vi "modbus_rtu.vi"() -> ()   [LabVIEW 2020]
uses:
  <vilib>/Plasmionique/MB Master/MB_Master/MB_Master.lvclass
  <vilib>/Plasmionique/MB Master/MB_ADU/MB_ADU.lvclass/MB_ADU.ctl
  <vilib>/Plasmionique/MB Master/MB_ADU/Read TX Data.vi
  <vilib>/Plasmionique/MB Master/MB_ADU/Read RX Data.vi
  <vilib>/Plasmionique/MB Master/MB_ADU/Read RX Timestamp.vi
  <vilib>/Plasmionique/MB Master/MB_Master_Serial/MB_Master_Serial.lvclass
  C:/Program Files/National Instruments/LabVIEW 2020/vi.lib/Plasmionique/MB Master/MB_Master/MB_Master.lvclass
  <vilib>/Plasmionique/MB Master/MB_ADU/MB_ADU.lvclass
  <vilib>/Plasmionique/MB Master/MB Master.lvlib
panel:
  in  "Tab Control 2":enum32{"Comm Settings", "Comm Status"}(tab)
  in  "Open":bool
  in  "Close":bool
  in  "Poll Period (ms)":i32=100
  in  "COM Port":refnum<visa-resource-name>
  in  "Mode":enum16{"RTU", "ASCII"}(ring)
  in  "Slave Address":u8=1
  in  "Baud Rate (bps)":u32(ring)=19200 items=["9600"=9600, "19200"=19200, "38400"=38400, "57600"=57600, "115200"=115200, "460800"=460800, "921600"=921600]
  in  "Stop Bits":u16(ring)=10 items=["1.0"=10, "1.5"=15, "2.0"=20]
  in  "Parity":u16(ring) items=["None", "Odd", "Even", "Mark", "Space"]
  in  "Flow Control":u16(ring) items=["None", "XON/XOFF", "RTS/CTS", "XON/XOFF & RTS/CTS", "DTR/DSR", "XON/XOFF & DTR/DSR"]
  in  "Timeout (ms)":u32=300
  in  "Retries":i32=1
  out "Last Error Status":errorcluster
  out "Last RX":string
  out "Last TX":string
  out "Last RX Time":string
  out "Last Error Time":string
  out "dt (ms)":u32
  in  "IR Poll":bool
  in  "HR Poll":bool
  out "Open?":bool caption="Connected"
  in  "Write Hld Regs":bool
  in  "Read Hld Regs":bool
  in  "Read In Regs":bool
  in  "HR QTY":u16=1 caption="Quantity"
  in  "HR SA":u16 caption="Starting Address"
  in  "Holding Registers":u16[](array[numeric])
  in  "IR QTY":u16=1 caption="Quantity"
  in  "IR SA":u16 caption="Starting Address"
  out "Input Registers":u16[](array[numeric])
  # "Communication Settngs"
  # "Communication Status"
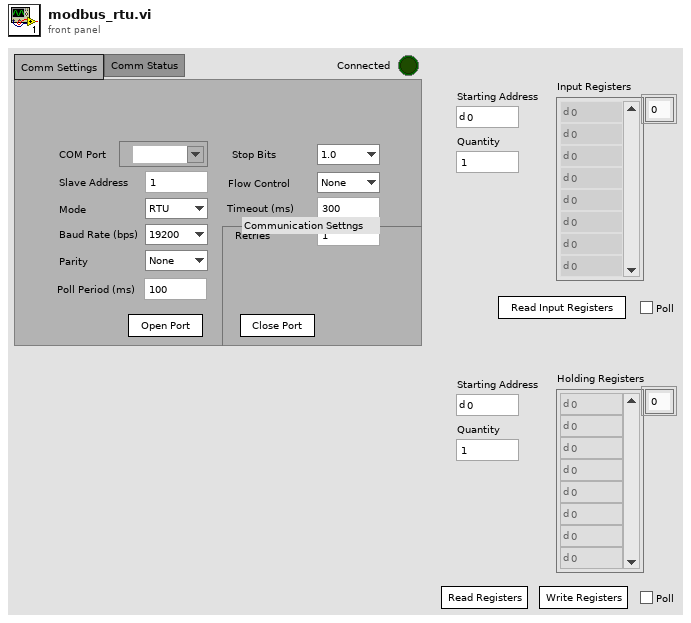
[diagram p1: front panel]
types:
  T1 = cluster{"baud rate (bps)":u32, "stop bits":u16, "parity":u16, "flow control":u16, "timeout":u32, "retries":i32}
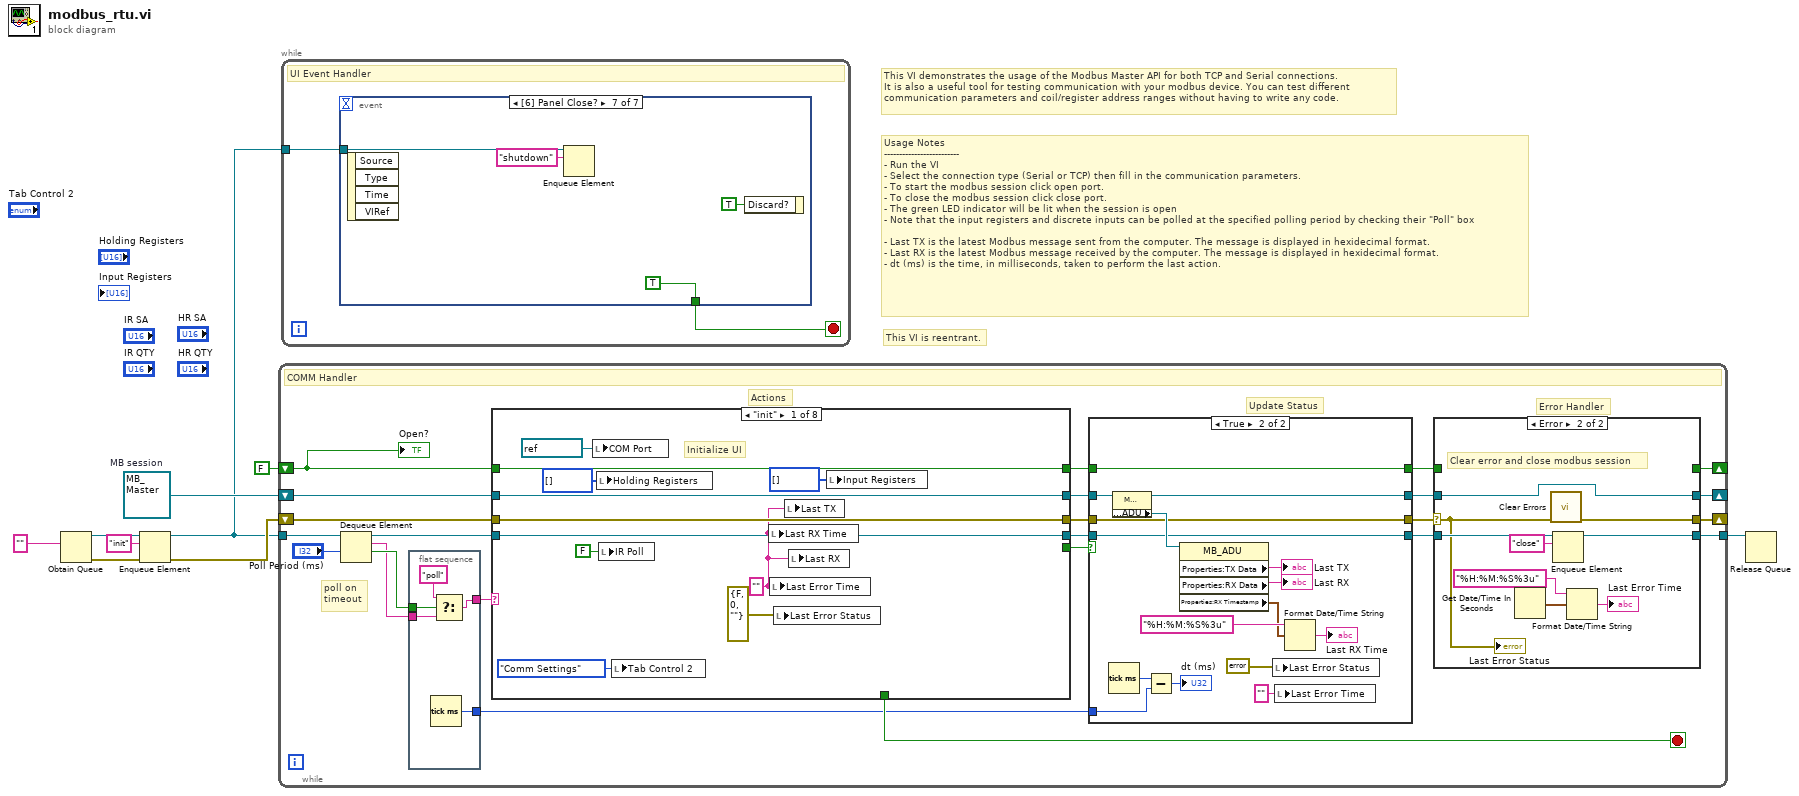
[diagram p0: block diagram]
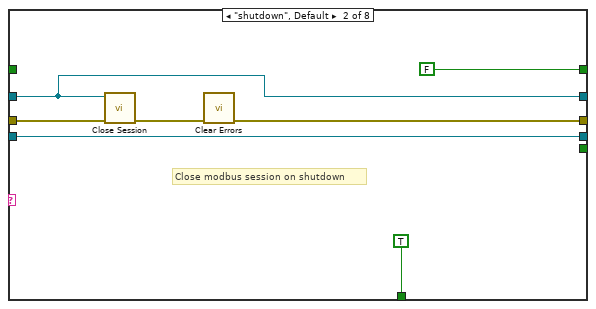
[diagram p4: hidden frame]
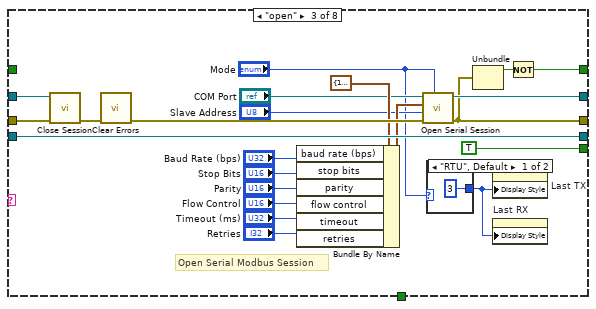
[diagram p5: hidden frame]
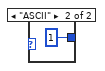
[diagram p6: hidden frame]
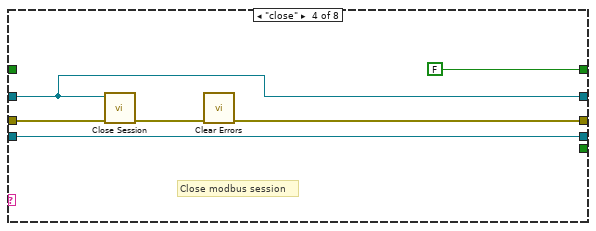
[diagram p7: hidden frame]
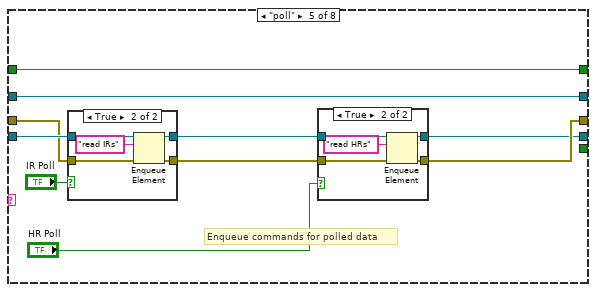
[diagram p8: hidden frame]
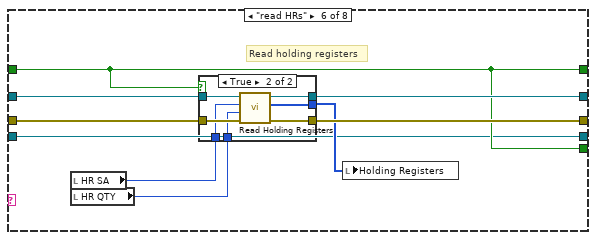
[diagram p11: hidden frame]
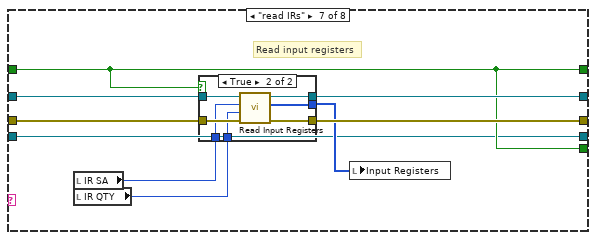
[diagram p13: hidden frame]
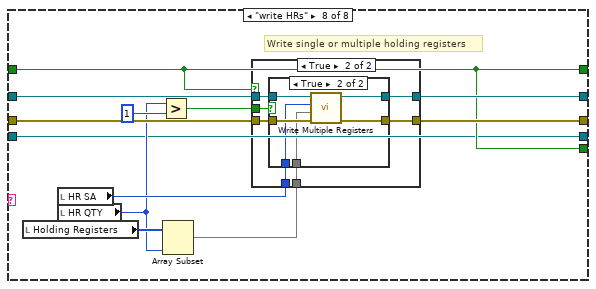
[diagram p15: hidden frame]
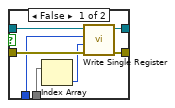
[diagram p17: hidden frame]
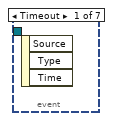
[diagram p18: hidden frame]
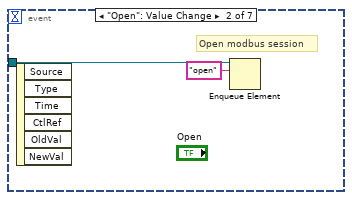
[diagram p19: hidden frame]
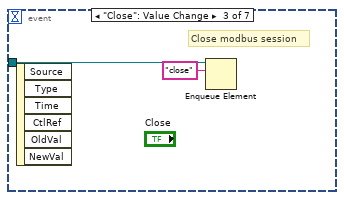
[diagram p20: hidden frame]
diagram:
  w7 = refnum<class "MB_Master.lvclass"> refnum  # MB session
  # "This VI is reentrant."
  # "Usage Notes\n-------------------------\n- Run the VI\n- Select the connection type (Serial or TCP) then fill in the communication parameters.\n- To start the modbus session click open port.\n- To close the modbus session click close port.\n- The green LED indicator will be lit when the session is open\n- Note that the input registers and discrete inputs can be polled at the specified polling period by checking their \"Poll\" box\n\n- Last TX is the latest Modbus message sent from the computer. The message is displayed in hexidecimal format.\n- Last RX is the latest Modbus message received by the computer. The message is displayed in hexidecimal format. \n- dt (ms) is the time, in milliseconds, taken to perform the last action."
  # "This VI demonstrates the usage of the Modbus Master API for both TCP and Serial connections.\nIt is also a useful tool for testing communication with your modbus device. You can test different\ncommunication parameters and coil/register address ranges without having to write any code."
  n1 = Obtain Queue(element data type="") -> (queue out=w6:refnum<queue>, error out=w4:errorcluster)  [unwired: 4 in, 1 out]
  n2 = Enqueue Element(queue=w6, element="init", error in (no error)=w4) -> (queue out=w2:refnum<queue>, error out=w3:errorcluster)  [unwired: 1 in, 1 out]
  n3 = while {
    tunnel: w2 -> [w33]
    shift-right: [w16] -> _
    shift-left: w7 -> [w32]
    shift-right: [w23] -> _
    shift-left: w3 -> [w24]
    shift-right: [w18] -> _
    shift-left: FALSE -> [w28]
    tunnel: [w22] -> w1
    stop <- w31 stop-if-true
    # "poll on\ntimeout"
    # "Actions"
    # "Error Handler"
    # "Update Status"
    # "COMM Handler"
    n4 = Dequeue Element(queue=w33, timeout in ms (-1)="Poll Period (ms)") -> (queue out=w30:refnum<queue>, element=w20:string, timed out?=w21:bool)  [unwired: 1 in, 1 out]
    n5 = flat-sequence {
      tunnel: [w51] -> w25
      tunnel: w21 -> [w50]
      tunnel: w20 -> [w49]
      tunnel: [w47] -> w19
      frame #0 {
        n6 = Tick Count (ms)() -> (millisecond timer value=w51:u32)
        n7 = Select(t="poll", s=w50, f=w49) -> (s? t:f=w47:string)
      }
    }
    n8 = case shown="\"init\"" w19 {
      tunnel: [w81 w86 w111 w116 w125 w150 w168 w188] -> w29
      tunnel: w32 -> [w81 w86 w106 w116 w125 w152 w170 w191]
      tunnel: [w80 w87 w110 w117 w123 w149 w167 w186] -> w13
      tunnel: w24 -> [w80 w89 w105 w119 w127 w151 w169 w187]
      tunnel: [_ TRUE _ _ _ _ _ _] -> w31
      tunnel: w30 -> [w74 w83 w103 w114 w128 w144 w162 w180]
      tunnel: w28 -> [w78 _ _ _ w126 w145 w163 w181]
      tunnel: [w78 FALSE w109 FALSE w126 w145 w163 w181] -> w15
      tunnel: [_ _ TRUE _ _ w145 w163 w181] -> w27
      tunnel: [w74 w83 w103 w114 w122 w144 w162 w180] -> w11
      frame "init" {
        w79 = "" ("Last Error Time")
        # "Initialize UI"
        n9 = local write "COM Port"(refnum<visa-resource-name> refnum ("COM Port")) -> ()
        n10 = local write "Holding Registers"(u16[] [] ("Holding Registers")) -> ()
        n11 = local write "IR Poll"(FALSE ("IR Poll")) -> ()
        n12 = local write "Tab Control 2"(enum32{"Comm Settings", "Comm Status"}."Comm Settings" ("Tab Control 2")) -> ()
        n13 = local write "Last RX Time"(w79) -> ()
        n14 = local write "Last Error Time"(w79) -> ()
        n15 = local write "Last Error Status"(errorcluster {"status"=FALSE, "code"=0, "source"=""} ("Last Error Status")) -> ()
        n16 = local write "Last TX"(w79) -> ()
        n17 = local write "Last RX"(w79) -> ()
        n18 = local write "Input Registers"(u16[] [] ("Input Registers")) -> ()
      }
      frame "shutdown", Default {
        # "Close modbus session on shutdown"
        n19 = call-dynamic "Close Session.vi"("error in (no error)"=w89, "MB session in"=w86) -> ("error out"=w88:errorcluster)  [unwired: 9 in]
        n20 = call <vilib>:"Clear Errors.vi"("error in (no error)"=w88) -> ("error out"=w87:errorcluster)  [unwired: 5 in, 1 out]
      }
      frame "open" {
        # "Open Serial Modbus Session"
        n21 = call-dynamic "Close Session.vi"("error in (no error)"=w105, "MB session in"=w106) -> ("error out"=w107:errorcluster)  [unwired: 9 in]
        n22 = call <vilib>:"Clear Errors.vi"("error in (no error)"=w107) -> ("error out"=w104:errorcluster)  [unwired: 5 in, 1 out]
        n23 = Bundle By Name(cluster=T1 {"baud rate (bps)"=19200, "stop bits"=10, "parity"=0, "flow control"=0, "timeout"=1000, "retries"=1} ("Serial Config"), "baud rate (bps)"="Baud Rate (bps)", "stop bits"="Stop Bits", "parity"="Parity", "flow control"="Flow Control", "timeout"="Timeout (ms)", "retries"="Retries") -> (w94:T1)
        n24 = call <vilib>:"Open Serial Session.vi"("Mode (RTU)"="Mode", "Error in"=w104, "Slave ID"="Slave Address", "Serial Config"=w94, "VISA Resource"="COM Port") -> ("Error out"=w110:errorcluster, "MB_Serial session"=w111:refnum<class "MB_Master_Serial.lvclass">)  [unwired: 5 in]
        n25 = case shown="\"RTU\", Default" "Mode" {
          tunnel: [u32 3 ("Display Style") u32 1 ("Display Style")] -> w90
          frame "RTU", Default {
          }
          frame "ASCII" {
          }
        }
        n26 = Unbundle(w110) -> ("status"=w92:bool)  [unwired: 2 out]
        n27 = property on="Last TX" class="Str"("Display Style"=w90) -> ()  [unwired: 2 in, 2 out]
        n28 = property on="Last RX" class="Str"("Display Style"=w90) -> ()  [unwired: 2 in, 2 out]
        n29 = Not(x=w92) -> (.not. x?=w109:bool)
      }
      frame "close" {
        # "Close modbus session"
        n30 = call-dynamic "Close Session.vi"("error in (no error)"=w119, "MB session in"=w116) -> ("error out"=w118:errorcluster)  [unwired: 9 in]
        n31 = call <vilib>:"Clear Errors.vi"("error in (no error)"=w118) -> ("error out"=w117:errorcluster)  [unwired: 5 in, 1 out]
      }
      frame "poll" {
        # "Enqueue commands for polled data"
        n32 = case shown="True" "IR Poll" {
          tunnel: w128 -> [w138 w142]
          tunnel: [w138 w141] -> w120
          tunnel: w127 -> [w137 w140]
          tunnel: [w137 w139] -> w121
          frame False {
          }
          frame True {
            n33 = Enqueue Element(queue=w142, element="read IRs", error in (no error)=w140) -> (queue out=w141:refnum<queue>, error out=w139:errorcluster)  [unwired: 1 in, 1 out]
          }
        }
        n34 = case shown="True" "HR Poll" {
          tunnel: w120 -> [w130 w135]
          tunnel: w121 -> [w131 w134]
          tunnel: [w131 w133] -> w123
          tunnel: [w130 w132] -> w122
          frame False {
          }
          frame True {
            n35 = Enqueue Element(queue=w135, element="read HRs", error in (no error)=w134) -> (queue out=w132:refnum<queue>, error out=w133:errorcluster)  [unwired: 1 in, 1 out]
          }
        }
      }
      frame "read HRs" {
        # "Read holding registers"
        n36 = local read "HR SA"() -> (w147:u16)
        n37 = local read "HR QTY"() -> (w146:u16)
        n38 = case shown="True" w145 {
          tunnel: w152 -> [w154 w161]
          tunnel: w151 -> [w153 w160]
          tunnel: [w154 w159] -> w150
          tunnel: [w153 w158] -> w149
          tunnel: w147 -> [_ w157]
          tunnel: w146 -> [_ w156]
          tunnel: [_ w155] -> w148
          frame False {
          }
          frame True {
            n39 = call <vilib>:"Read Holding Registers.vi"("error in (no error)"=w160, "quantity"=w156, "starting address"=w157, "MB session in"=w161) -> ("error out"=w158:errorcluster, "Registers"=w155:u16[], "MB session out"=w159:refnum<class "MB_Master.lvclass">)  [unwired: 5 in]
          }
        }
        n40 = local write "Holding Registers"(w148) -> ()
      }
      frame "read IRs" {
        # "Read input registers"
        n41 = local read "IR SA"() -> (w165:u16)
        n42 = local read "IR QTY"() -> (w164:u16)
        n43 = case shown="True" w163 {
          tunnel: w170 -> [w172 w179]
          tunnel: w169 -> [w171 w178]
          tunnel: [w172 w177] -> w168
          tunnel: [w171 w176] -> w167
          tunnel: w165 -> [_ w175]
          tunnel: w164 -> [_ w174]
          tunnel: [_ w173] -> w166
          frame False {
          }
          frame True {
            n44 = call <vilib>:"Read Input Registers.vi"("error in (no error)"=w178, "quantity"=w174, "starting address"=w175, "MB session in"=w179) -> ("error out"=w176:errorcluster, "Registers"=w173:u16[], "MB session out"=w177:refnum<class "MB_Master.lvclass">)  [unwired: 5 in]
          }
        }
        n45 = local write "Input Registers"(w166) -> ()
      }
      frame "write HRs" {
        # "Write single or multiple holding registers"
        n46 = local read "Holding Registers"() -> (w184:u16[])
        n47 = local read "HR SA"() -> (w185:u16)
        n48 = local read "HR QTY"() -> (w183:u16)
        n49 = Greater?(x=w183, y=u16 1) -> (0:w189:bool)
        n50 = Array Subset(array=w184, length=w183) -> (w182:u16[])  [unwired: 1 in]
        n51 = case shown="True" w181 {
          tunnel: w191 -> [w193 w200]
          tunnel: w189 -> [_ w199]
          tunnel: [w193 w198] -> w188
          tunnel: w187 -> [w192 w197]
          tunnel: [w192 w196] -> w186
          tunnel: w185 -> [_ w195]
          tunnel: w182 -> [_ w194]
          frame False {
          }
          frame True {
            n52 = case shown="True" w199 {
              tunnel: w200 -> [w207 w213]
              tunnel: [w201 w212] -> w198
              tunnel: w197 -> [w206 w211]
              tunnel: [w202 w210] -> w196
              tunnel: w195 -> [w205 w209]
              tunnel: w194 -> [w204 w208]
              frame False {
                n53 = Index Array(array=w204) -> (element=w203:u16)  [unwired: 1 in]
                n54 = call <vilib>:"Write Single Register.vi"("error in (no error)"=w206, "value"=w203, "address"=w205, "MB session in"=w207) -> ("error out"=w202:errorcluster, "MB session out"=w201:refnum<class "MB_Master.lvclass">)  [unwired: 6 in]
              }
              frame True {
                n55 = call <vilib>:"Write Multiple Registers.vi"("error in (no error)"=w211, "values"=w208, "starting address"=w209, "MB session in"=w213) -> ("error out"=w210:errorcluster, "MB session out"=w212:refnum<class "MB_Master.lvclass">)  [unwired: 6 in]
              }
            }
          }
        }
      }
    }
    n56 = case shown="True" w27 {
      tunnel: w29 -> [w55 w56]
      tunnel: [w55 w69] -> w17
      tunnel: w25 -> [_ w63]
      tunnel: w15 -> [w54 w59]
      tunnel: [w54 w59] -> w14
      tunnel: w13 -> [w53 w58]
      tunnel: [w53 w58] -> w12
      tunnel: w11 -> [w52 w57]
      tunnel: [w52 w57] -> w10
      frame False {
      }
      frame True {
        n57 = Tick Count (ms)() -> (millisecond timer value=w62:u32)
        n58 = property class="MB_Master"(reference=w56) -> (reference out=w69:refnum<class "MB_Master.lvclass">, "Properties:ADU"=w70:refnum<class "MB_ADU.lvclass">)  [unwired: 1 in, 1 out]
        n59 = Subtract(x=w62, y=w63) -> (x-y=→"dt (ms)":u32)
        n60 = property class="MB_ADU"(reference=w70) -> ("Properties:TX Data"=→"Last TX":string, "Properties:RX Data"=→"Last RX":string, "Properties:RX Timestamp"=w60:timestamp)  [unwired: 1 in, 2 out]
        n61 = local write "Last Error Status"(errorcluster {"status"=FALSE, "code"=0, "source"=""} ("Last Error Status")) -> ()
        n62 = local write "Last Error Time"("" ("Last Error Time")) -> ()
        n63 = Format Date/Time String(time format string (%c)="%H:%M:%S%3u", seconds (now)=w60) -> (date/time string=→"Last RX Time":string)  [unwired: 1 in]
      }
    }
    n64 = case shown="Error" w12 {
      selector: w12 -> [w37 w39]
      tunnel: [w37 w43] -> w23
      tunnel: w10 -> [w36 w41]
      tunnel: [w36 w40] -> w22
      tunnel: w14 -> [w35 _]
      tunnel: [w35 _] -> w18
      tunnel: w17 -> [w34 w38]
      tunnel: [w34 w38] -> w16
      frame No Error {
      }
      frame Error {
        # "Clear error and close modbus session"
        n65 = Get Date/Time In Seconds() -> (seconds since 1Jan1904=w44:timestamp)
        n66 = call <vilib>:"Clear Errors.vi"("error in (no error)"=w39) -> ("error out"=w43:errorcluster)  [unwired: 5 in, 1 out]
        n67 = Enqueue Element(queue=w41, element="close") -> (queue out=w40:refnum<queue>)  [unwired: 2 in, 2 out]
        n68 = Format Date/Time String(time format string (%c)="%H:%M:%S%3u", seconds (now)=w44) -> (date/time string=→"Last Error Time":string)  [unwired: 1 in]
        "Last Error Status" <- w39
      }
    }
    "Open?" <- w28
  }
  n69 = while {
    tunnel: w2 -> [w215]
    stop <- w214 stop-if-true
    # "UI Event Handler"
    n70 = event shown="[6] Panel Close?" {
      selector: _ -> [_ _ _ _ _ _ _]
      dyn-events: _ -> [_ _ _ _ _ _ _]
      timeout: _ -> [_ _ _ _ _ _ _]
      tunnel: w215 -> [_ w217 w218 w220 w222 w224 w226]
      tunnel: [_ _ _ _ _ _ TRUE] -> w214
      event Timeout {
        n71 = event-data() -> ()  [unwired: 1 in, 3 out]
      }
      event "Open": Value Change {
        # "Open modbus session"
        n72 = event-data() -> ()  [unwired: 1 in, 6 out]
        n73 = Enqueue Element(queue=w217, element="open") -> ()  [unwired: 2 in, 3 out]
      }
      event "Close": Value Change {
        # "Close modbus session"
        n74 = event-data() -> ()  [unwired: 1 in, 6 out]
        n75 = Enqueue Element(queue=w218, element="close") -> ()  [unwired: 2 in, 3 out]
      }
      event "Read In Regs": Value Change {
        n76 = event-data() -> ()  [unwired: 1 in, 6 out]
        n77 = Enqueue Element(queue=w220, element="read IRs") -> ()  [unwired: 2 in, 3 out]
      }
      event "Read Hld Regs": Value Change {
        n78 = event-data() -> ()  [unwired: 1 in, 6 out]
        n79 = Enqueue Element(queue=w222, element="read HRs") -> ()  [unwired: 2 in, 3 out]
      }
      event "Write Hld Regs": Value Change {
        n80 = event-data() -> ()  [unwired: 1 in, 6 out]
        n81 = Enqueue Element(queue=w224, element="write HRs") -> ()  [unwired: 2 in, 3 out]
      }
      event Panel Close? {
        n82 = event-data() -> ()  [unwired: 1 in, 4 out]
        n83 = Enqueue Element(queue=w226, element="shutdown") -> ()  [unwired: 2 in, 3 out]
        n84 = event-data("Discard?"=TRUE) -> ()  [unwired: 1 in, 1 out]
      }
    }
  }
  n85 = Release Queue(queue=w1) -> ()  [unwired: 2 in, 3 out]
